vi "Load File.vi"(8 "error in (no error)":errorcluster, 10 "File Path":path, 11 "Data Loader in":refnum<class "Data Loader.lvclass">) -> (0 "error out":errorcluster, 3 "Data Loader out":refnum<class "Data Loader.lvclass">)   [LabVIEW 2020, in "Data Loader.lvlib" / "Data Loader.lvclass"]
uses:
  Data Loader.lvclass
  Data Loader.lvclass/Data Loader.ctl
  Data Types/Abstrut Data/Abstruct Data Type.lvclass/Abstruct Data Type.ctl
  Data Types/Abstrut Data/Accessors/Write File Path.vi
  Accessor/Write File Path.vi
  Accessor/Read Data.vi
  Accessor/Read Data File.lvclass.vi
  Accessor/Write Data.vi
  Accessor/Write Data File.lvclass.vi
  Data Types/Abstrut Data/Abstruct Data Type.lvclass
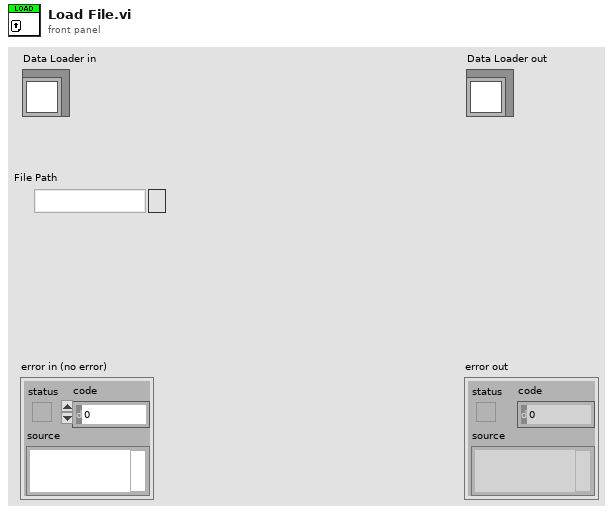
[diagram p1: front panel]
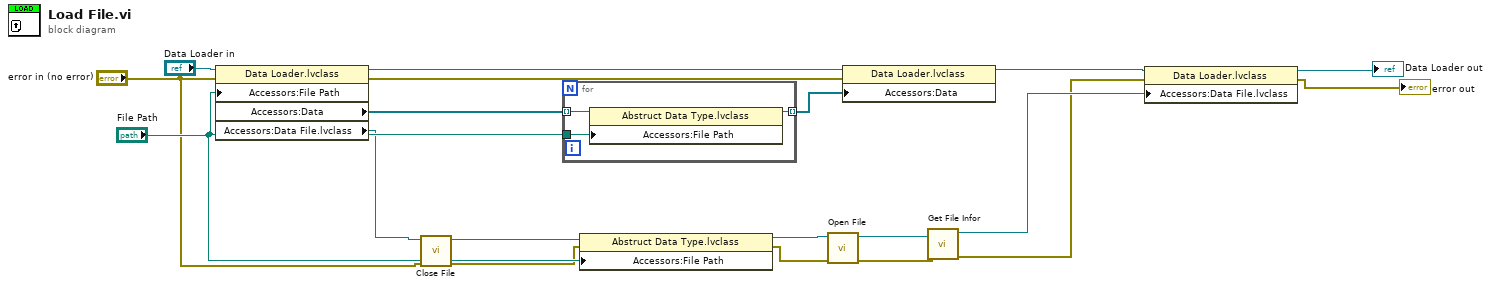
[diagram p0: block diagram]
diagram:
  n1 = property class="Data Loader.lvclass"(reference="Data Loader in", error in="error in (no error)", "Accessors:File Path"="File Path") -> (reference out=w17:refnum<class "Data Loader.lvclass">, error out=w15:errorcluster, "Accessors:Data"=w18:refnum<class "Abstruct Data Type.lvclass">[], "Accessors:Data File.lvclass"=w4:refnum<class "Abstruct Data Type.lvclass">)
  n2 = call-dynamic "Close File.vi"("error in (no error)"="error in (no error)", "Abstruct Data Type in"=w4) -> ("error out"=w2:errorcluster, "Abstruct Data Type out"=w3:refnum<class "Abstruct Data Type.lvclass">)  [unwired: 8 in]
  n3 = for {
    tunnel: w18 -> [w22] mode=indexing
    tunnel: "File Path" -> [w21]
    tunnel: [w20] -> w16 mode=indexing
    n4 = property class="Abstruct Data Type.lvclass"(reference=w22, "Accessors:File Path"=w21) -> (reference out=w20:refnum<class "Abstruct Data Type.lvclass">)  [unwired: 1 in, 1 out]
  }
  n5 = property class="Abstruct Data Type.lvclass"(reference=w3, error in=w2, "Accessors:File Path"="File Path") -> (reference out=w13:refnum<class "Abstruct Data Type.lvclass">, error out=w12:errorcluster)
  n6 = call-dynamic "Open File.vi"("error in (no error)"=w12, "Abstruct Data Type in"=w13) -> ("error out"=w10:errorcluster, "Abstruct Data Type out"=w11:refnum<class "Abstruct Data Type.lvclass">)  [unwired: 8 in]
  n7 = property class="Data Loader.lvclass"(reference=w17, error in=w15, "Accessors:Data"=w16) -> (reference out=w9:refnum<class "Data Loader.lvclass">)  [unwired: 1 out]
  n8 = call-dynamic "Get File Infor.vi"("error in (no error)"=w10, "Abstruct Data Type in"=w11) -> ("error out"=w5:errorcluster, "Abstruct Data Type out"=w6:refnum<class "Abstruct Data Type.lvclass">)  [unwired: 8 in]
  n9 = property class="Data Loader.lvclass"(reference=w9, error in=w5, "Accessors:Data File.lvclass"=w6) -> (reference out=→"Data Loader out":refnum<class "Data Loader.lvclass">, error out=→"error out":errorcluster)
